vi "NI_FPGA_PPG.set pdc interval.vi"(0 "i ref in":refnum<vi>, 2 "enable_pdc":bool, 3 "ms timeout (10000)":i32=10000, 5 "error in (no error)":errorcluster) -> (14 "i ref out":refnum<vi>, 17 "timed out":bool, 19 "error out":errorcluster)   [LabVIEW 2014, in "NI_FPGA_PPG.lvlib"]
doc: "special method for handling the interval of the periodic loop"
uses:
  NI_FPGA_PPG.lvlib
  CS_Core/CSSystem/CoreLib/CoreLib.int 2 byte array.vi
  CS_Core/CSSystem/CoreLib/CoreLib.lvlib
  CS_Core/CSSystem/CSSystemLib/CSSystemLib.lvlib
  CS_Core/BaseProcess/BaseProcess.lvlib
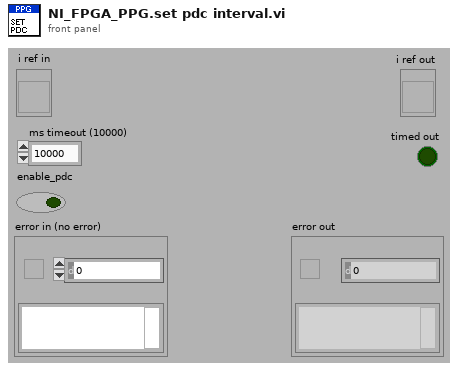
[diagram p1: front panel]
types:
  T1 = typedef "NI_FPGA_PPG.lvlib/NI_FPGA_PPG.i attribute.ctl" = cluster{"dim_service_id":cluster{"dim_actual_device_status":i32, "dim_event_data":i32, "dim_cmd_data":i32, "dim_cmd_data _description":i32, "dim_channel_description":i32}, "VISA":refnum<visa-resource-name>, "actual_device_status":i32, "event_data_id":i32, "pdc_enabled":bool, "pdc_timestamp":u32, "cmd_data_string":string, "cmd_data_size":i32, "cmd_data_description_string":string, "cmd_data_description_size":i32, "channel_description_string":string, "channel_description_size":i32}
  T2 = typedef "CoreDefs.rawDataType.ctl" = i8[]
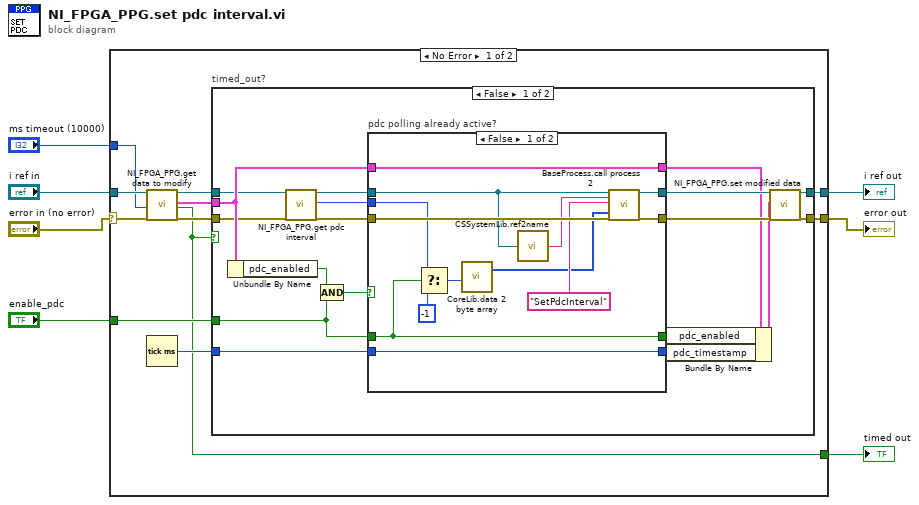
[diagram p0: block diagram]
diagram:
  n1 = case shown="No Error" "error in (no error)" {
    selector: "error in (no error)" -> [w16 w58]
    tunnel: "i ref in" -> [w17 w57]
    tunnel: [w10 w57] -> w5
    tunnel: [w9 w58] -> w4
    tunnel: "ms timeout (10000)" -> [w15 _]
    tunnel: "enable_pdc" -> [w18 _]
    tunnel: [w8 _] -> w1
    frame No Error {
      n2 = call "NI_FPGA_PPG.get data to modify.vi"("i ref in"=w17, "ms timeout (10000)"=w15, "error in (no error)"=w16) -> ("i ref out"=w12:refnum<vi>, "i attribute"=w13:T1, "timed out"=w8:bool, "error out"=w14:errorcluster)  [unwired: 13 in]
      n3 = Tick Count (ms)() -> (millisecond timer value=w11:u32)
      n4 = case "timed_out?" shown="False" w8 {
        tunnel: w18 -> [w35 _]
        tunnel: w14 -> [w26 w55]
        tunnel: w13 -> [w31 _]
        tunnel: w12 -> [w27 w56]
        tunnel: w11 -> [w30 _]
        tunnel: [w29 w56] -> w10
        tunnel: [w28 w55] -> w9
        frame False {
          n5 = Unbundle By Name(w31) -> ("pdc_enabled"=w36:bool)
          n6 = call "NI_FPGA_PPG.get pdc interval.vi"("i ref in"=w27, "error in (no error)"=w26) -> ("i ref out"=w25:refnum<vi>, "pdc_interval"=w23:i32, "error out"=w24:errorcluster)  [unwired: 15 in]
          n7 = Compound Arithmetic op=AND(w36, w35) -> (w34:bool)
          n8 = case "pdc polling already active?" shown="False" w34 {
            tunnel: w24 -> [w49 w53]
            tunnel: [w48 w54] -> w33
            tunnel: w25 -> [w45 w54]
            tunnel: [w43 w53] -> w32
            tunnel: w35 -> [w38 w51]
            tunnel: w31 -> [w39 w52]
            tunnel: w30 -> [w37 w50]
            tunnel: [w39 w52] -> w22
            tunnel: w23 -> [w40 _]
            tunnel: [w38 w51] -> w20
            tunnel: [w37 w50] -> w19
            frame False {
              n9 = Select(t=w40, s=w38, f=-1) -> (s? t:f=w42:i32)
              n10 = call-poly "CoreLib.data 2 byte array.vi"("i32"=w42) -> ("byteArray out"=w44:T2)  [unwired: 18 in]
              n11 = call "CSSystemLib.ref2name.vi"("obj refnum"=w45) -> ("name"=w47:string)
              n12 = call "BaseProcess.call process 2.vi"("i ref in"=w45, "Object"=w47, "Selector"="SetPdcInterval", "Data"=w44, "error in (no error)"=w49) -> ("i ref out"=w48:refnum<vi>, "error out"=w43:errorcluster)  [unwired: 13 in]
            }
            frame True {
            }
          }
          n13 = Bundle By Name(cluster=w22, "pdc_enabled"=w20, "pdc_timestamp"=w19) -> (w21:T1)
          n14 = call "NI_FPGA_PPG.set modified data.vi"("i ref in"=w33, "i attribute"=w21, "error in (no error)"=w32) -> ("i ref out"=w29:refnum<vi>, "error out"=w28:errorcluster)  [unwired: 15 in]
        }
        frame True {
        }
      }
    }
    frame Error {
    }
  }
  "error out" <- w4
  "timed out" <- w1
  "i ref out" <- w5
